vi "Class Child URL.vi"(7 "Destination":path=path "", 8 "Error In":errorcluster, 11 "Name":string) -> (0 "Error Out":errorcluster, 3 "Child URL":string)   [LabVIEW 2018, in "Scripts.lvlib"]
uses:
  Scripts.lvlib
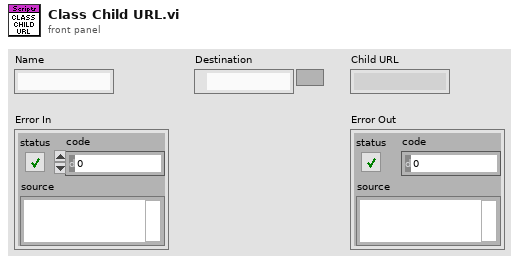
[diagram p1: front panel]
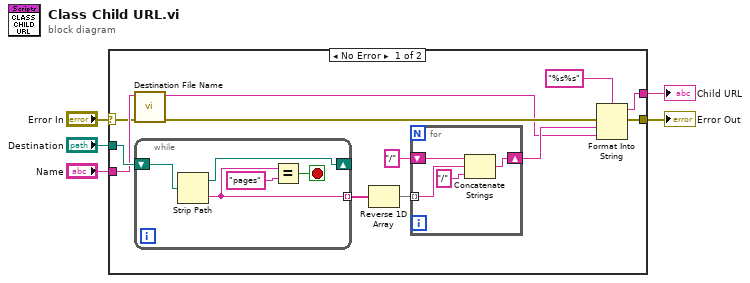
[diagram p0: block diagram]
diagram:
  n1 = case shown="No Error" "Error In" {
    selector: "Error In" -> [w6 w27]
    tunnel: [w16 w27] -> w5
    tunnel: [w15 _] -> w4
    tunnel: "Destination" -> [w14 _]
    tunnel: "Name" -> [w9 _]
    frame No Error {
      n2 = call "Destination File Name.vi"("Error In"=w6, "File Stem"=w9) -> ("Error Out"=w8:errorcluster, "Destination File Name"=w7:string)  [unwired: 8 in]
      n3 = while {
        shift-right: [w24] -> _
        shift-left: w14 -> [w25]
        tunnel: [w22] -> w10 mode=indexing
        stop <- w23 stop-if-true
        n4 = Strip Path(path=w25) -> (stripped path=w24:path, name=w22:string)
        n5 = Equal?(x=w22, y="pages") -> (x = y?=w23:bool)
      }
      n6 = Reverse 1D Array(array=w10) -> (reversed array=w13:string[])
      n7 = for {
        tunnel: w13 -> [w20] mode=indexing
        shift-right: [w18] -> w11
        shift-left: "/" -> [w21]
        n8 = Concatenate Strings(w21, w20, "/") -> (w18:string)
      }
      n9 = Format Into String(format string="%s%s", error in=w8, w11, w7) -> (resulting string=w15:string, error out=w16:errorcluster)  [unwired: 1 in]
    }
    frame Error {
    }
  }
  "Error Out" <- w5
  "Child URL" <- w4
